vi "Files Outside Folder.vi"(8 "error in (no error)":errorcluster, 10 "Folder":path, 11 "LVProject in":refnum<class "LVProject.lvclass">) -> (0 "error out":errorcluster, 2 "External Files":path[](array[path]), 3 "LVProject out":refnum<class "LVProject.lvclass">)   [LabVIEW 2020, in "GPack.lvlib" / "LVProject.lvclass"]
uses:
  LVProject.lvclass
  LVProject.lvclass/LVProject.ctl
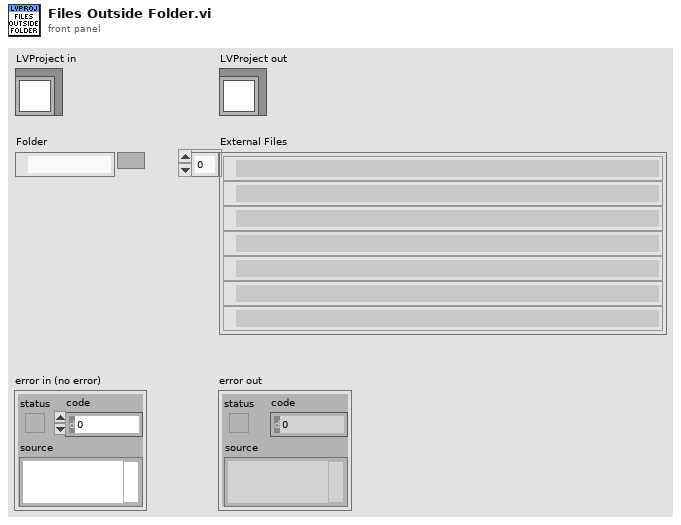
[diagram p1: front panel]
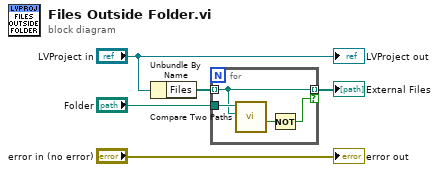
[diagram p0: block diagram]
diagram:
  n1 = Unbundle By Name("LVProject in") -> ("Files"=w3:path[])
  n2 = for {
    tunnel: w3 -> [w8] mode=indexing
    tunnel: "Folder" -> [w9]
    tunnel: [w8] -> w1 mode=indexing if=w6
    n3 = call <vilib>:"Compare Two Paths.vi"("Path 2"=w8, "Path 1"=w9) -> ("Path 2 Relative to Path 1?"=w7:bool)  [unwired: 6 in, 3 out]
    n4 = Not(x=w7) -> (.not. x?=w6:bool)
  }
  "External Files" <- w1
  "error out" <- "error in (no error)"
  "LVProject out" <- "LVProject in"
